vi "QX_AssignSignals.vi"(8 "Error in":errorcluster, 11 "DevRef[]":T1(array[cluster])) -> (0 "Error out":errorcluster)   [LabVIEW 2016]
doc: "Assigns the settings of the given signals to the physical signal of the according device."
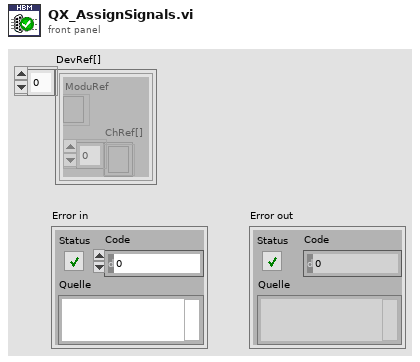
[diagram p1: front panel]
types:
  T1 = cluster{"ModuRef":refnum<k24>, "ChRef[]":refnum<k24>[]}[]
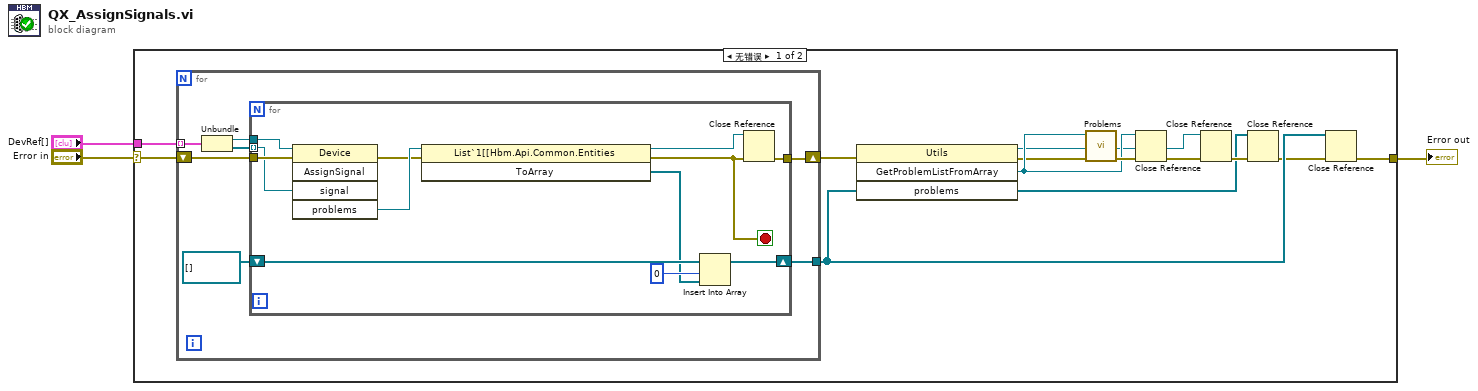
[diagram p0: block diagram]
diagram:
  n1 = case shown="无错误" "Error in" {
    selector: "Error in" -> [w15 w36]
    tunnel: [w5 w36] -> w3
    tunnel: "DevRef[]" -> [w4 _]
    frame No Error {
      n2 = for {
        tunnel: [w20] -> w9
        shift-right: [w22] -> w16
        shift-left: w15 -> [w21]
        tunnel: w4 -> [w19] mode=indexing
        n3 = Unbundle(w19) -> ("ModuRef"=w17:refnum<k24>, "ChRef[]"=w18:refnum<k24>[])
        n4 = for {
          tunnel: w21 -> [w26]
          shift-right: [w35] -> w20
          shift-left: refnum<k24>[] [] -> [w34]
          tunnel: [w28] -> w22
          tunnel: w18 -> [w24] mode=indexing
          tunnel: w17 -> [w25]
          stop <- w30 stop-if-true
          n5 = invoke on="Methodenknoten" class="Device" method="AssignSignal"(reference=w25, error in=w26, "signal"=w24) -> (error out=w31:errorcluster, "problems"=w32:refnum<k24>)  [unwired: 2 in, 3 out]
          n6 = invoke on="Methodenknoten" class="List`1[[Hbm.Api.Common.Entities" method="ToArray"(reference=w32, error in=w31) -> (reference out=w29:refnum<k24>, error out=w30:errorcluster, "ToArray"=w27:refnum<k24>[])  [unwired: 1 in]
          n7 = Insert Into Array(array=w34, index=0 ("Index"), new element=w27) -> (w35:refnum<k24>[])
          n8 = Close Reference(reference=w29, error in (no error)=w30) -> (error out=w28:errorcluster)
        }
      }
      n9 = invoke on="Methodenknoten" class="Utils" method="GetProblemListFromArray"(error in=w16, "problems"=w9) -> (reference out=w11:refnum<k24>, error out=w10:errorcluster, "GetProblemListFromArray"=w13:refnum<k24>, "problems"=w6:refnum<k24>[])  [unwired: 2 in]
      n10 = call "Problems.vi"("Error in"=w10, "Problems"=w13) -> ("Error out"=w14:errorcluster)  [unwired: 9 in]
      n11 = Close Reference(reference=w13, error in (no error)=w14) -> (error out=w12:errorcluster)
      n12 = Close Reference(reference=w11, error in (no error)=w12) -> (error out=w7:errorcluster)
      n13 = Close Reference(reference=w6, error in (no error)=w7) -> (error out=w8:errorcluster)
      n14 = Close Reference(reference=w9, error in (no error)=w8) -> (error out=w5:errorcluster)
    }
    frame Error {
    }
  }
  "Error out" <- w3
